vi "Plot Helper.vi"   [LabVIEW 2017, in "3D Bar Datatype.lvclass"]
doc: "Generates a plot of vertical bars."
uses:
  <vilib>/Math Plots/3D Math Plots/3D Bar/3D Bar Datatype/3D Bar Datatype.lvclass
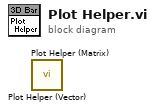
[diagram p0: block diagram]
diagram:
  n1 = call <vilib>:"Plot Helper (Vector).vi"() -> ()  [unwired: 10 in, 2 out]
  n2 = call <vilib>:"Plot Helper (Matrix).vi"() -> ()  [unwired: 10 in, 2 out]
